vi "读取固件状态.vi"(8 "错误输入":errorcluster, 11 "MB session in":refnum<class "MB_Master.lvclass">) -> (0 "error out":errorcluster, 2 "结果字符串":string, 3 "MB session out":refnum<class "MB_Master.lvclass">)   [LabVIEW 2016]
uses:
  <vilib>/Plasmionique/MB Master/MB_Master/MB_Master.lvclass
  <vilib>/Plasmionique/MB Master/MB_Master_Serial/MB_Master_Serial.lvclass
  D:/Program Files (x86)/National Instruments/LabVIEW 2016/vi.lib/Plasmionique/MB Master/MB_Master/MB_Master.lvclass
  <vilib>/Plasmionique/MB Master/MB Master.lvlib
panel:
  in  "VISA Resource":refnum<visa-resource-name>
  in  "引用选择":enum16{"MB引用", "自建引用"}(ring)
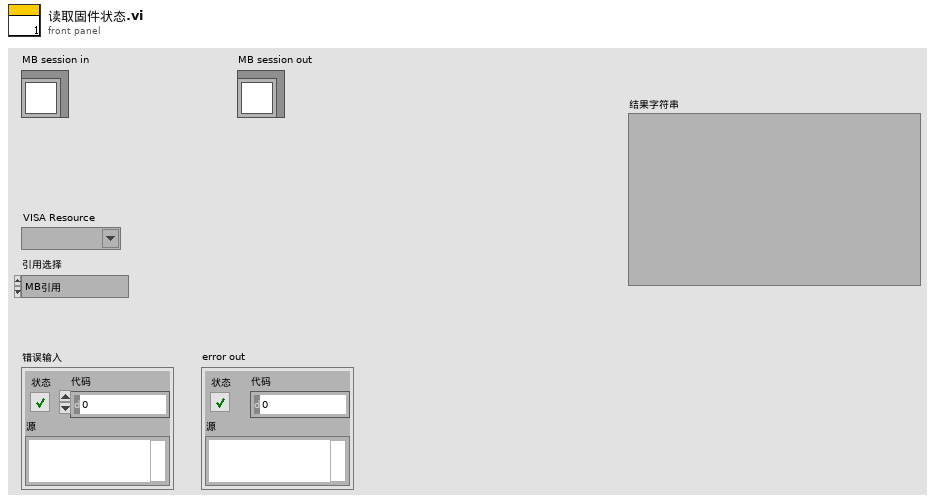
[diagram p1: front panel]
types:
  T1 = cluster{"baud rate (bps)":u32, "stop bits":u16, "parity":u16, "flow control":u16, "timeout":u32, "retries":i32}
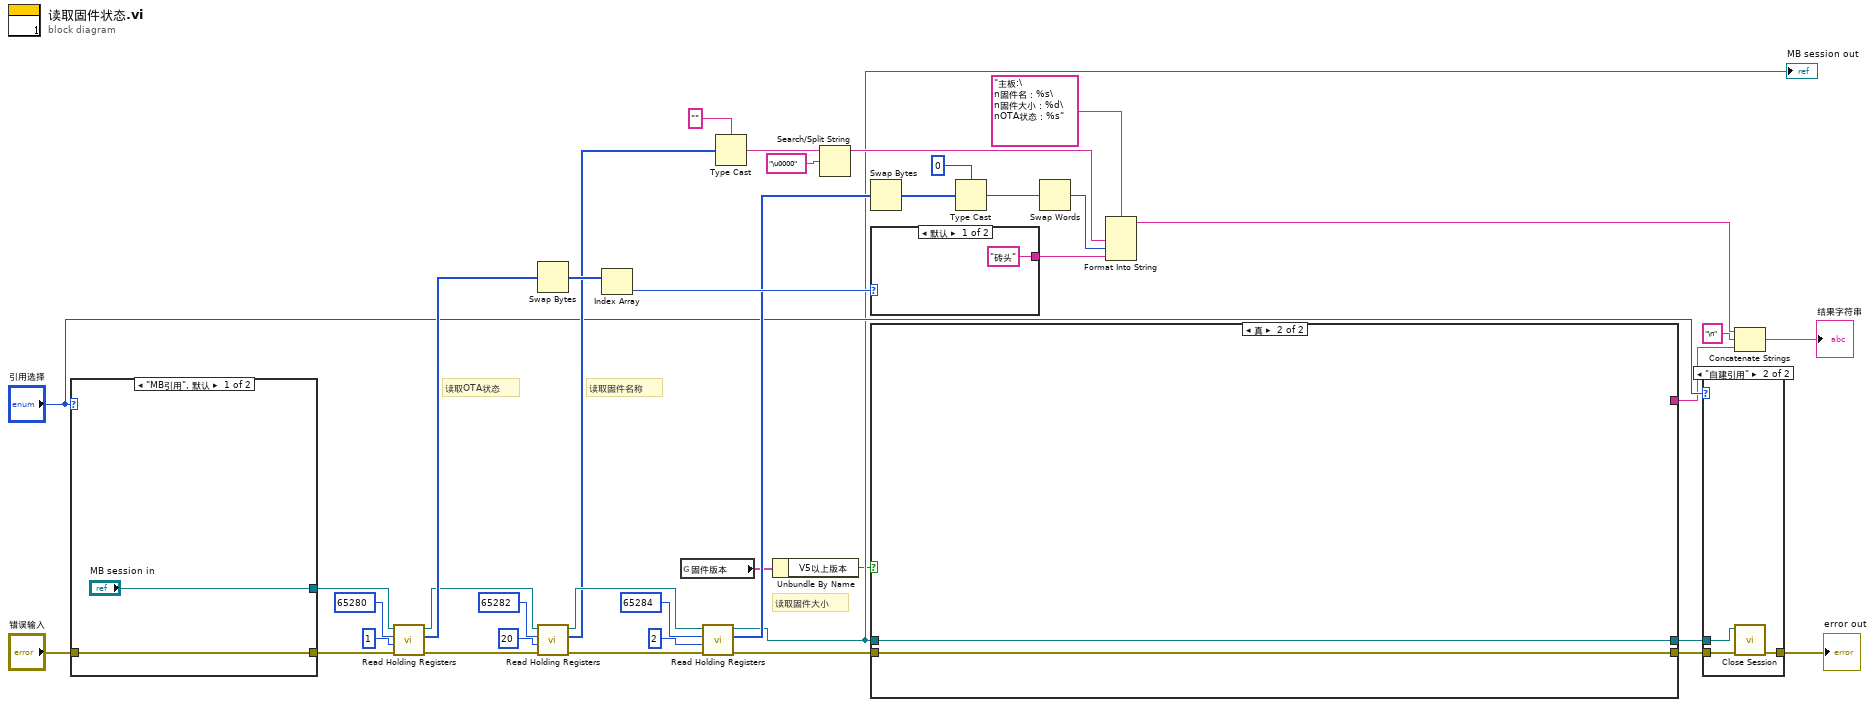
[diagram p0: block diagram]
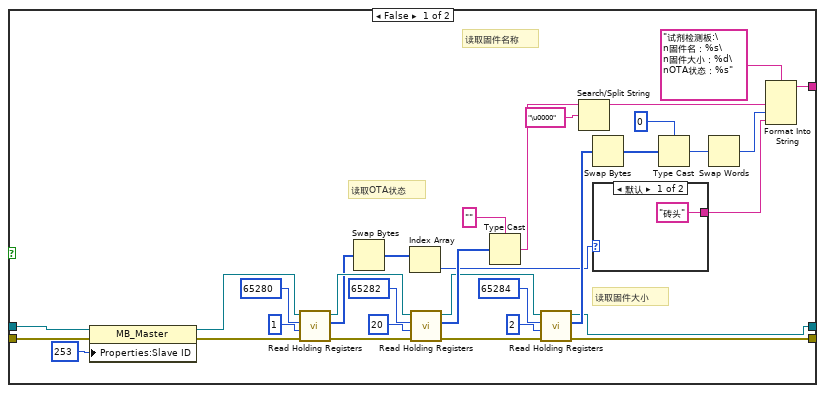
[diagram p2: hidden frame]
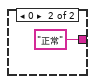
[diagram p3: hidden frame]
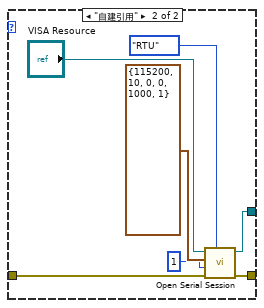
[diagram p5: hidden frame]
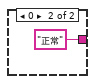
[diagram p6: hidden frame]
diagram:
  # "读取固件大小"
  # "读取固件名称"
  # "读取OTA状态"
  n1 = case shown="\"MB引用\", 默认" "引用选择" {
    tunnel: ["MB session in" w48] -> w39
    tunnel: "错误输入" -> [w41 w47]
    tunnel: [w41 w46] -> w19
    frame "MB引用", Default {
    }
    frame "自建引用" {
      n2 = call <vilib>:"Open Serial Session.vi"("Mode (RTU)"=enum16{"RTU", "ASCII"}."RTU", "Error in"=w47, "Slave ID"=u8 1, "Serial Config"=T1 {"baud rate (bps)"=115200, "stop bits"=10, "parity"=0, "flow control"=0, "timeout"=1000, "retries"=1}, "VISA Resource"="VISA Resource") -> ("Error out"=w46:errorcluster, "MB_Serial session"=w48:refnum<class "MB_Master_Serial.lvclass">)  [unwired: 5 in]
    }
  }
  n3 = call <vilib>:"Read Holding Registers.vi"("error in (no error)"=w19, "quantity"=u16 1, "starting address"=u16 65280, "MB session in"=w39) -> ("error out"=w27:errorcluster, "Registers"=w36:u16[], "MB session out"=w32:refnum<class "MB_Master.lvclass">)  [unwired: 5 in]
  n4 = Swap Bytes(anything=w36) -> (byte swapped=w34:u16[])
  n5 = call <vilib>:"Read Holding Registers.vi"("error in (no error)"=w27, "quantity"=u16 20, "starting address"=u16 65282, "MB session in"=w32) -> ("error out"=w26:errorcluster, "Registers"=w13:u16[], "MB session out"=w30:refnum<class "MB_Master.lvclass">)  [unwired: 5 in]
  n6 = Index Array(array=w34) -> (element=w35:u16)  [unwired: 1 in]
  n7 = global read "VAR挥发酚全局变量.vi" "固件版本"() -> (w2:cluster{"V5以上版本":bool, "版本号":dbl})
  n8 = call <vilib>:"Read Holding Registers.vi"("error in (no error)"=w26, "quantity"=u16 2, "starting address"=u16 65284, "MB session in"=w30) -> ("error out"=w5:errorcluster, "Registers"=w25:u16[], "MB session out"=w6:refnum<class "MB_Master.lvclass">)  [unwired: 5 in]
  "MB session out" <- w6
  n9 = Type Cast(type="", x=w13) -> (*(type *) &x=w14:string)
  n10 = Unbundle By Name(w2) -> ("V5以上版本"=w1:bool)
  n11 = Search/Split String(string=w14, search string/char (-)="\u0000" ("搜索字符串")) -> (substring before match=w16:string)  [unwired: 1 in, 2 out]
  n12 = Swap Bytes(anything=w25) -> (byte swapped=w24:u16[])
  n13 = case shown="默认" w35 {
    tunnel: ["砖头" "正常"] -> w33
    frame Default {
    }
    frame 0 {
    }
  }
  n14 = case shown="真" w1 {
    tunnel: [w59 w88] -> w8
    tunnel: [w58 w87] -> w7
    tunnel: w6 -> [w57 w88]
    tunnel: w5 -> [w53 w87]
    tunnel: [w52 _] -> w3
    frame False {
      # "读取固件大小"
      # "读取固件名称"
      # "读取OTA状态"
      n15 = property class="MB_Master"(reference=w57, error in=w53, "Properties:Slave ID"=u8 253 ("Slave ID")) -> (reference out=w55:refnum<class "MB_Master.lvclass">, error out=w54:errorcluster)
      n16 = call <vilib>:"Read Holding Registers.vi"("error in (no error)"=w54, "quantity"=u16 1, "starting address"=u16 65280, "MB session in"=w55) -> ("error out"=w73:errorcluster, "Registers"=w65:u16[], "MB session out"=w68:refnum<class "MB_Master.lvclass">)  [unwired: 5 in]
      n17 = Swap Bytes(anything=w65) -> (byte swapped=w67:u16[])
      n18 = Index Array(array=w67) -> (element=w66:u16)  [unwired: 1 in]
      n19 = call <vilib>:"Read Holding Registers.vi"("error in (no error)"=w73, "quantity"=u16 20, "starting address"=u16 65282, "MB session in"=w68) -> ("error out"=w74:errorcluster, "Registers"=w83:u16[], "MB session out"=w70:refnum<class "MB_Master.lvclass">)  [unwired: 5 in]
      n20 = Type Cast(type="", x=w83) -> (*(type *) &x=w82:string)
      n21 = call <vilib>:"Read Holding Registers.vi"("error in (no error)"=w74, "quantity"=u16 2, "starting address"=u16 65284, "MB session in"=w70) -> ("error out"=w58:errorcluster, "Registers"=w75:u16[], "MB session out"=w59:refnum<class "MB_Master.lvclass">)  [unwired: 5 in]
      n22 = Search/Split String(string=w82, search string/char (-)="\u0000" ("搜索字符串")) -> (substring before match=w60:string)  [unwired: 1 in, 2 out]
      n23 = Swap Bytes(anything=w75) -> (byte swapped=w76:u16[])
      n24 = case shown="默认" w66 {
        tunnel: ["砖头" "正常"] -> w62
        frame Default {
        }
        frame 0 {
        }
      }
      n25 = Type Cast(type=u32 0, x=w76) -> (*(type *) &x=w78:u32)
      n26 = Swap Words(1:w78) -> (0:w61:u32)
      n27 = Format Into String(format string="试剂检测板:\n固件名：%s\n固件大小：%d\nOTA状态：%s" ("格式字符串"), w60, w61, w62) -> (resulting string=w52:string)  [unwired: 2 in, 1 out]
    }
    frame True {
    }
  }
  n28 = Type Cast(type=u32 0, x=w24) -> (*(type *) &x=w22:u32)
  n29 = Swap Words(1:w22) -> (0:w21:u32)
  n30 = Format Into String(format string="主板:\n固件名：%s\n固件大小：%d\nOTA状态：%s" ("格式字符串"), w16, w21, w33) -> (resulting string=w10:string)  [unwired: 2 in, 1 out]
  n31 = case shown="\"自建引用\"" "引用选择" {
    tunnel: w8 -> [_ w92]
    tunnel: w7 -> [w89 w91]
    tunnel: [w89 w90] -> w9
    frame "MB引用", Default {
    }
    frame "自建引用" {
      n32 = call-dynamic "Close Session.vi"("error in (no error)"=w91, "MB session in"=w92) -> ("error out"=w90:errorcluster)  [unwired: 9 in]
    }
  }
  "error out" <- w9
  n33 = Concatenate Strings(w10, "\n", w3) -> (→"结果字符串":string)
